vi "Get Current Time Structure.vi"(0 "Use Mountain Standard Time":bool) -> (1 "current local time":timestamp=timestamp(3531623303.360785 s since 1904-01-01), 4 "Y":i32=2015, 6 "M":i32=11, 8 "Day with fraction":dbl=29.269714814814815, 12 "Hour":i32=6, 13 "Minute":i32=28, 14 "Second":i32=23, 15 "Fractional Second":dbl=0.36)   [LabVIEW 2015]
panel:
  out "Fractional Day":dbl=0.2697148148148148
  out "D":i32=29
  # "Mountain Standard Time is Universal Coordinated Time (UTC) - 7 Hours"
  # "These fractional day calculations are based on UTC (not local time)"
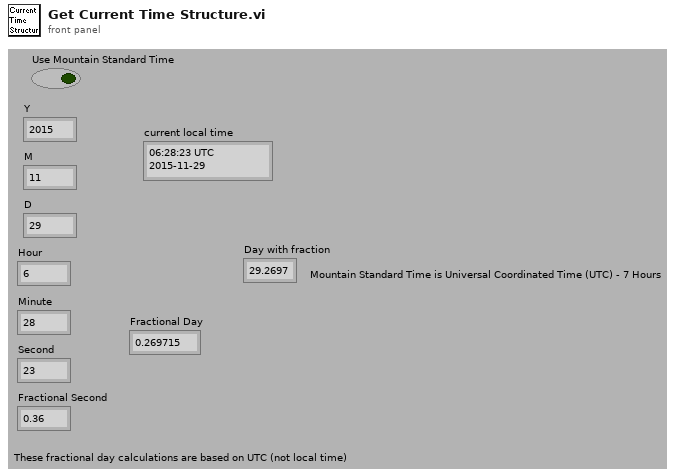
[diagram p1: front panel]
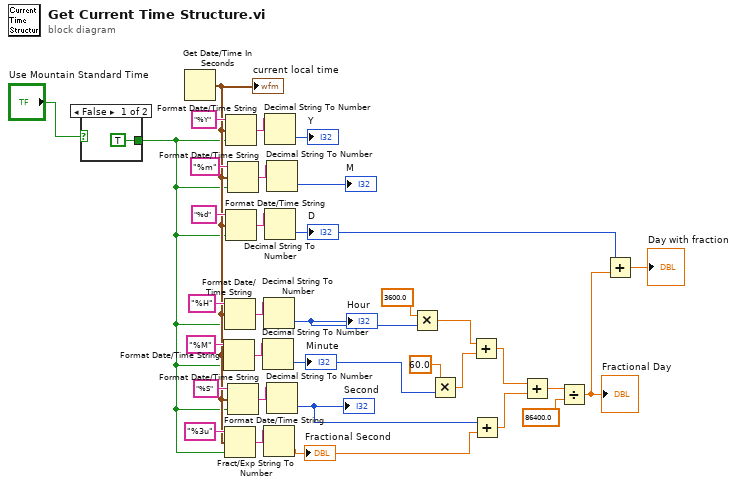
[diagram p0: block diagram]
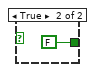
[diagram p2: hidden frame]
diagram:
  n1 = case shown="False" "Use Mountain Standard Time" {
    tunnel: [TRUE ("UTC format") FALSE ("UTC format")] -> w2
    frame False {
    }
    frame True {
    }
  }
  n2 = Get Date/Time In Seconds() -> (seconds since 1Jan1904=w18:timestamp)
  "current local time" <- w18
  n3 = Format Date/Time String(time format string (%c)="%M", seconds (now)=w18, UTC format=w2) -> (date/time string=w23:string)
  n4 = Format Date/Time String(time format string (%c)="%H", seconds (now)=w18, UTC format=w2) -> (date/time string=w25:string)
  n5 = Format Date/Time String(time format string (%c)="%3u", seconds (now)=w18, UTC format=w2) -> (date/time string=w19:string)
  n6 = Format Date/Time String(time format string (%c)="%Y", seconds (now)=w18, UTC format=w2) -> (date/time string=w33:string)
  n7 = Format Date/Time String(time format string (%c)="%d", seconds (now)=w18, UTC format=w2) -> (date/time string=w28:string)
  n8 = Format Date/Time String(time format string (%c)="%m", seconds (now)=w18, UTC format=w2) -> (date/time string=w30:string)
  n9 = Format Date/Time String(time format string (%c)="%S", seconds (now)=w18, UTC format=w2) -> (date/time string=w21:string)
  n10 = Decimal String To Number(string=w23) -> (number=w14:i32)  [unwired: 3 out]
  "Minute" <- w14
  n11 = Decimal String To Number(string=w25) -> (number=w16:i32)  [unwired: 3 out]
  "Hour" <- w16
  n12 = Fract/Exp String To Number(string=w19) -> (number=w9:dbl)  [unwired: 4 out]
  "Fractional Second" <- w9
  n13 = Decimal String To Number(string=w33) -> (number=→"Y":i32)  [unwired: 3 out]
  n14 = Decimal String To Number(string=w28) -> (number=w6:i32)  [unwired: 3 out]
  "D" <- w6
  n15 = Decimal String To Number(string=w30) -> (number=→"M":i32)  [unwired: 3 out]
  n16 = Decimal String To Number(string=w21) -> (number=w10:i32)  [unwired: 3 out]
  "Second" <- w10
  n17 = Multiply(x=3600.0, y=w16) -> (x*y=w13:dbl)
  n18 = Multiply(x=60.0, y=w14) -> (x*y=w12:dbl)
  n19 = Add(x=w13, y=w12) -> (x+y=w11:dbl)
  n20 = Add(x=w10, y=w9) -> (x+y=w3:dbl)
  n21 = Add(x=w11, y=w3) -> (x+y=w8:dbl)
  n22 = Divide(x=w8, y=86400.0) -> (x/y=w5:dbl)
  "Fractional Day" <- w5
  n23 = Add(x=w6, y=w5) -> (x+y=→"Day with fraction":dbl)
